vi "Set Greeter_res.vi"(7 "Complete Call (T)":bool=TRUE, 8 "error in (no error)":errorcluster, 10 "package_templatemessage":T1, 11 "gRPCid":T2) -> (0 "error out":errorcluster)   [LabVIEW 2019, in "Generated_server.lvlib"]
uses:
  Generated_server.lvlib
  <vilib>/gRPC/LabVIEW gRPC Library/Shared/grpcId.ctl
  Greeter_res.ctl
  Greeter_res_res_oneof/Greeter_res_res_oneof.lvclass
  Greeter_res_Flat.ctl
  Greeter_res_res_oneof/Greeter_res_res_oneof.lvclass/Greeter_res_res_oneof.ctl
  dcc74a39-081a-4bdd-860b-8ed792803c96.vi
  Greeter_res_res_oneof/GetActiveFieldIndex.vi
  Greeter_res_res_oneof/Getres_int32.vi
  Greeter_res_res_oneof/Getres_int64.vi
  Greeter_res_res_oneof/Getres_uint32.vi
  Greeter_res_res_oneof/Getres_uint64.vi
  Greeter_res_res_oneof/Getres_sint32.vi
  Greeter_res_res_oneof/Getres_sint64.vi
  Greeter_res_res_oneof/Getres_fixed32.vi
  Greeter_res_res_oneof/Getres_fixed64.vi
  Greeter_res_res_oneof/Getres_sfixed32.vi
  Greeter_res_res_oneof/Getres_sfixed64.vi
  Greeter_res_res_oneof/Getres_float.vi
  Greeter_res_res_oneof/Getres_double.vi
  Greeter_res_res_oneof/Getres_bool.vi
  Greeter_res_res_oneof/Getres_string.vi
  Greeter_res_res_oneof/Getres_bytes.vi
  <vilib>/gRPC/LabVIEW gRPC Library/Shared/TranslateGrpcError.vi
  <vilib>/gRPC/LabVIEW gRPC Library/Server API/Server/Get Server DLL Path.vi
  <vilib>/Utility/error.llb/Error Cluster From Error Code.vi
  <vilib>/Utility/error.llb/Simple Error Handler.vi
  <vilib>/gRPC/LabVIEW gRPC Library/grpc-lvsupport-release.lvlib
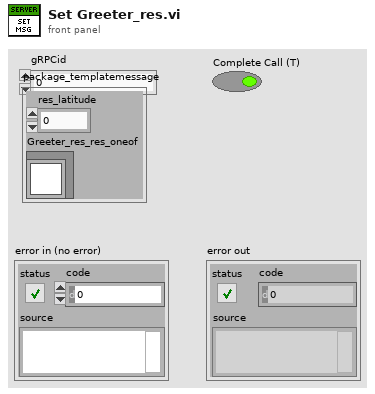
[diagram p1: front panel]
types:
  T1 = typedef "Generated_server.lvlib/Greeter_res.ctl" = cluster{"res_latitude":i32, "Greeter_res_res_oneof":refnum<class "Greeter_res_res_oneof.lvclass">}
  T2 = typedef "grpc-lvsupport-release.lvlib/grpcId.ctl" = u64
  T3 = typedef "Generated_server.lvlib/Greeter_res_Flat.ctl" = cluster{"res_latitude":i32, "Greeter_res_res_oneof_selected_index":i32, "res_int32":i32, "res_int64":i64, "res_uint32":u32, "res_uint64":u64, "res_sint32":i32, "res_sint64":i64, "res_fixed32":u32, "res_fixed64":u64, "res_sfixed32":i32, "res_sfixed64":i64, "res_float":sgl, "res_double":dbl, "res_bool":bool, "res_string":string, "res_bytes":u8[]}
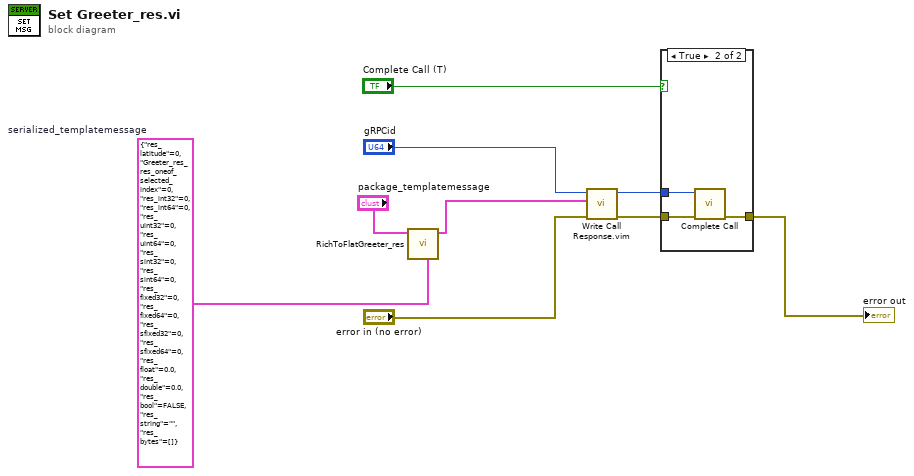
[diagram p0: block diagram]
diagram:
  w2 = T3 {"res_latitude"=0, "Greeter_res_res_oneof_selected_index"=0, "res_int32"=0, "res_int64"=0, "res_uint32"=0, "res_uint64"=0, "res_sint32"=0, "res_sint64"=0, "res_fixed32"=0, "res_fixed64"=0, "res_sfixed32"=0, "res_sfixed64"=0, "res_float"=0.0, "res_double"=0.0, "res_bool"=FALSE, "res_string"="", "res_bytes"=[]}  # serialized_templatemessage
  n1 = call "RichToFlatGreeter_res.vi"("OutputClusterType"=w2, "InputCluster"="package_templatemessage") -> ("OutputCluster"=w1:T3)  [unwired: 9 in]
  n2 = call "Write Call Response.vim"("error in"="error in (no error)", "Response Data"=w1, "gRPCid in"="gRPCid") -> ("error out"=w6:errorcluster, "gRPCid out"=w7:T2)  [unwired: 7 in]
  n3 = case shown="True" "Complete Call (T)" {
    tunnel: [w10 w13] -> w9
    tunnel: w7 -> [_ w12]
    tunnel: w6 -> [w10 w11]
    frame False {
    }
    frame True {
      n4 = call <vilib>:"Complete Call.vi"("gRPCid"=w12, "error in"=w11) -> ("error out"=w13:errorcluster)  [unwired: 8 in]
    }
  }
  "error out" <- w9
